vi "MS SQL_Read_80Count.vi"(0 "Ref in":T4, 1 "PokaYoke?":bool, 2 "Message":refnum<vi>, 11 "error in (no error)":errorcluster, 12 "Date Code":string) -> (3 "Pokayoke Done?":bool, 4 "Ref Out":T4, 8 "Routing":bool, 10 "Pky Status":T3, 14 "OPx PKYK Status":T1[](array[typedef]), 15 "error out":errorcluster)   [LabVIEW 2020]
uses:
  <vilib>/addons/database/Connection.llb/Conn ObjectReference.ctl
  <vilib>/addons/database/NI_Database_API.lvlib
  Controls/TD SQL.ctl
  Controls/Poka_Status.ctl
  Controls/PKYK_Status.ctl
  Controls/PKYK_Barcode_Status.ctl
  Controls/WIP_State.ctl
panel:
  out "resulting string":string
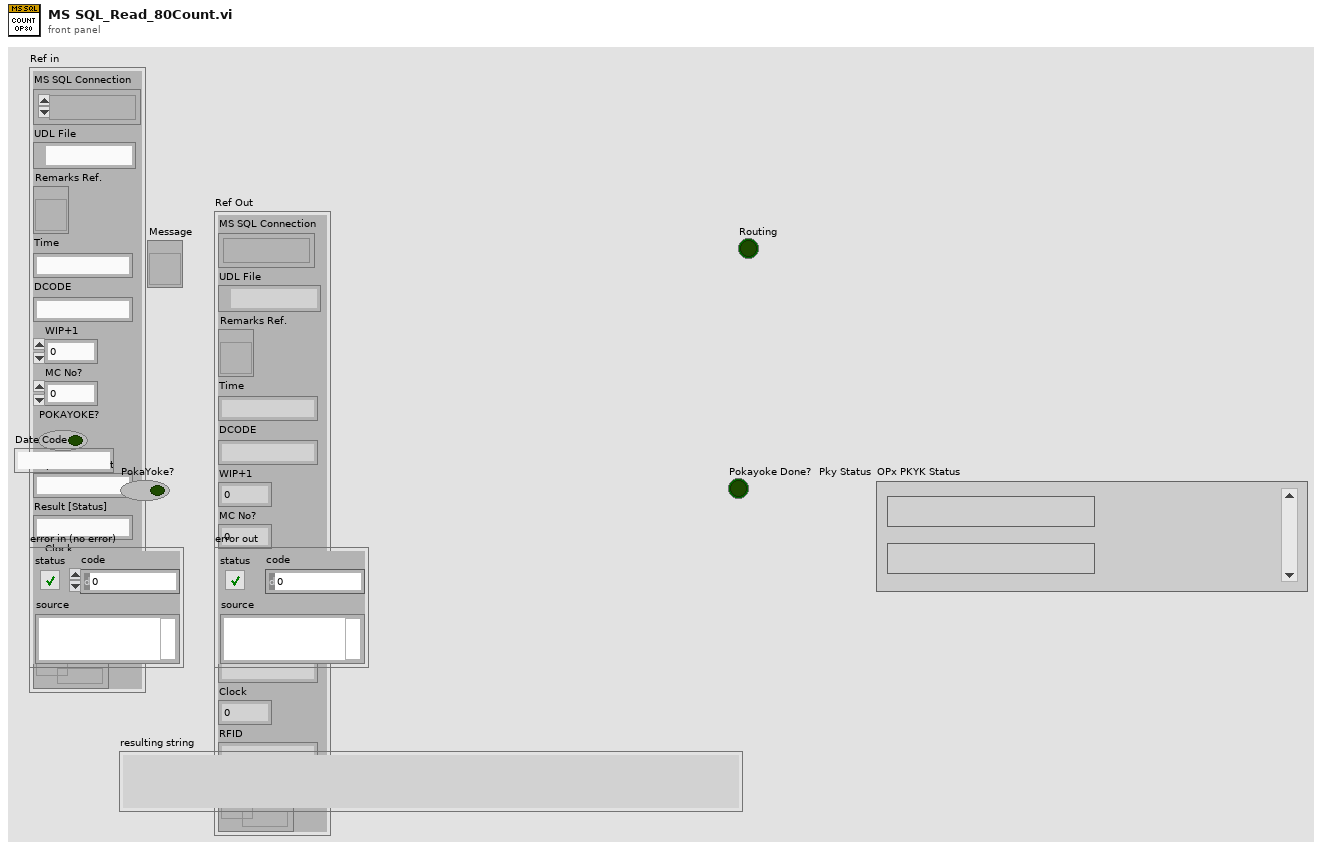
[diagram p1: front panel]
types:
  T1 = typedef "PKYK_Barcode_Status.ctl" = cluster{"RFID Written Last":string, "Result":T2, "Exp. Result":T2}
  T2 = typedef "PKYK_Status.ctl" = u16
  T3 = typedef "Poka_Status.ctl" = u16
  T4 = typedef "TD SQL.ctl" = cluster{"MS SQL Connection":T5, "UDL File":path, "Remarks Ref.":refnum<vi>, "Time":string, "DCODE":string, "WIP+1":i64, "MC No?":i32, "POKAYOKE?":bool, "Expected Result":string, "Result [Status]":string, "Clock":dbl, "RFID":string, "WIP Queue":refnum<queue>}
  T5 = typedef "NI_Database_API.lvlib/Conn ObjectReference.ctl" = refnum<k1>
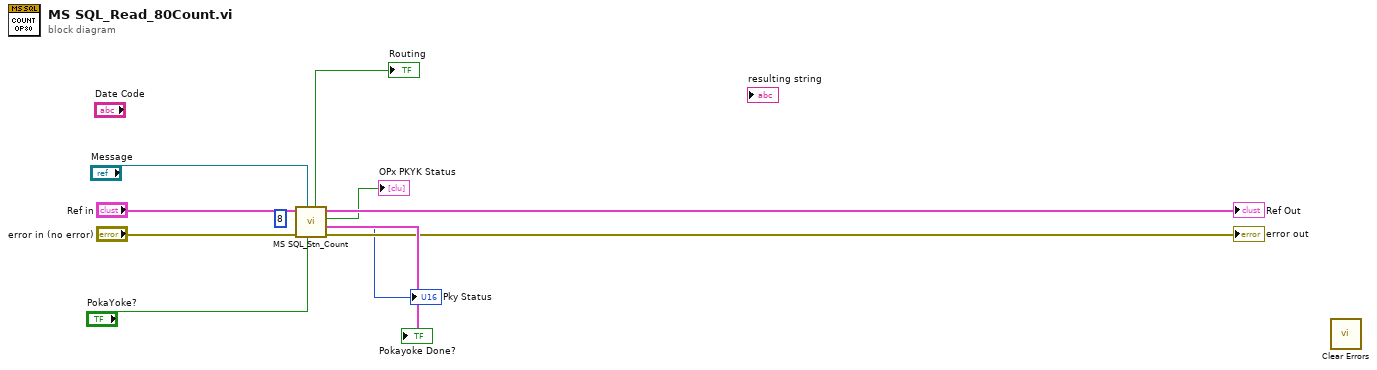
[diagram p0: block diagram]
diagram:
  (unwired) 8 ("Machine No")
  n1 = call "MS SQL_Stn_Count.vi"("Message"="PokaYoke?", 7:"Message", "error in (no error)"="error in (no error)", "Ref in"="Ref in") -> ("error out"=→"error out":errorcluster, "Pky Status"=→"Pky Status":T3, "Routing"=→"OPx PKYK Status":bool, "Ref Out"=→"Ref Out":T4, "OPx PKYK Status"=→"Pokayoke Done?":T1[], "Pokayoke Done?"=→"Routing":bool)  [unwired: 2 in]
  n2 = call <vilib>:"Clear Errors.vi"() -> ()  [unwired: 6 in, 2 out]
